vi "PH_ImageOperator.calc width diameter.vi"(7 "Best Fit Order":i32, 8 "Percent":dbl, 13 "Best Fit Width Parameter":dbl) -> (2 "Result":dbl)   [LabVIEW 2014, in "PH_ImageOperator.lvlib"]
doc: "This VI calculates from a Gaussian function of \"Best Fit Order\" with the \"Best Fit Parameter\" the width of wanted \"Percent\":\n\nResult = 2*(ln(\"Percent\"^(-1)))^(1/(2*\"Order\"))*\"Best Fit Width Parameter\""
uses:
  PH_ImageOperator.lvlib
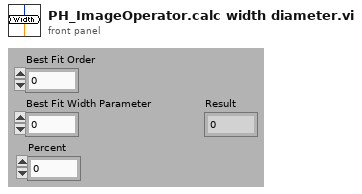
[diagram p1: front panel]
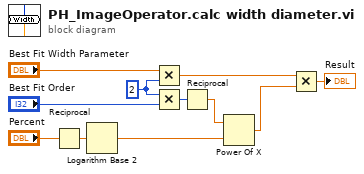
[diagram p0: block diagram]
diagram:
  w5 = 2
  n1 = Reciprocal(x="Percent") -> (1/x=w8:dbl)
  n2 = Logarithm Base 2(1:w8) -> (0:w7:dbl)
  n3 = Multiply(x="Best Fit Width Parameter", y=w5) -> (x*y=w10:dbl)
  n4 = Multiply(x=w5, y="Best Fit Order") -> (x*y=w4:i32)
  n5 = Reciprocal(x=w4) -> (1/x=w3:dbl)
  n6 = Power Of X(1:w7, 2:w3) -> (0:w2:dbl)
  n7 = Multiply(x=w10, y=w2) -> (x*y=→"Result":dbl)
